vi "Consumer.vi"(8 "error in (no error)":errorcluster, 9 "Data":variant, 10 "Case ID":string, 11 "Guardian Subpanel in":refnum<class "Guardian Subpanel.lvclass">) -> (0 "error out":errorcluster, 3 "Guardian Subpanel out":refnum<class "Guardian Subpanel.lvclass">)   [LabVIEW 2026, in "TALOS.lvlib" / "Guardian Subpanel.lvlib" / "Guardian Subpanel.lvclass"]
uses:
  Guardian Subpanel.lvclass
  C:/LabVIEW Code/TALOS/talos/Father of all uServices/Father of all uServices/Father of all uServices.lvclass
  Guardian Subpanel Consumer Case Selector.ctl
  <vilib>/Utility/error.llb/DialogType.ctl
  Father of all uServices/Father of all uServices/Father of all uServices.lvclass/Father of all uServices.ctl
  Ancestor/Ancestor/Ancestor.lvclass/Ancestor.ctl
  <vilib>/AdvancedString/1D String Array to Delimited String (string).vi
  Support VIs/Substitute Error.vi
  Support VIs/Generate Error.vi
  FGV/Error Memory/Get Error Description.vi
  Support VIs/Get PC name.vi
  Ancestor/Ancestor/Read ID.vi
  Support VIs/Get Class Name.vi
  FGV/Error Memory/Error Memory Core.vi
  <vilib>/AdvancedString/Delimited String to 1D String Array.vi
  <vilib>/AdvancedString/Delimited String to 1D String Array (string).vi
  FGV/Error Memory/Error Crt Lvl checker.vi
  FGV/Error Memory/Error Memory Core.vi/40c8088d-b597-4017-91af-faa98e00292e.vi
  FGV/Error Memory/Error Memory Core.vi/d4a3ab98-063c-4e44-b43d-fbdcfe6c2be2.vi
  Support VIs/Global Memory.vi
  <vilib>/Utility/LVClass/Get LV Class Name.vi
  Support VIs/Is in Packed Library.vi
  Support VIs/TALOS Root path.vi
  Support VIs/Read CSV worksheet.vi
  Support VIs/Global Constants.vi
  <vilib>/Utility/error.llb/General Error Handler.vi
  Support VIs/Error Log.vi
  Ancestor/Ancestor/Ancestor.lvclass
  <vilib>/Comparison/Equal/Equal Functor/Equal Functor.lvclass
  Father of all uServices/Father of all uServices/Father of all uServices.lvclass
  TALOS.lvlib
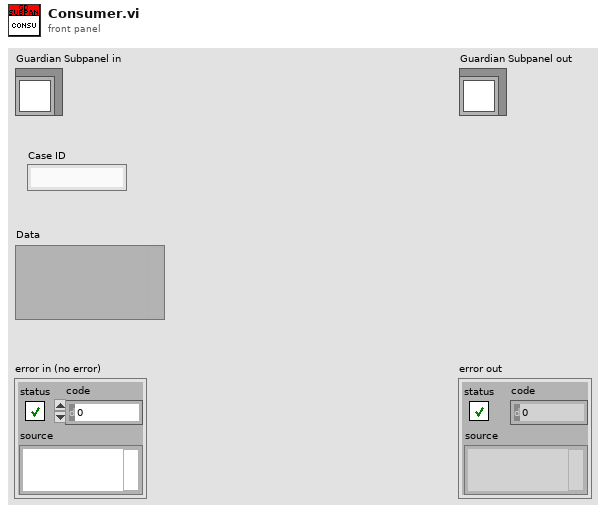
[diagram p1: front panel]
types:
  T1 = typedef "TALOS.lvlib/Guardian Subpanel.lvlib/Guardian Subpanel.lvclass/Guardian Subpanel Consumer Case Selector.ctl" = enum16{"uServices launchable", "Update Bearer"}
  T2 = typedef "DialogType.ctl" = u16
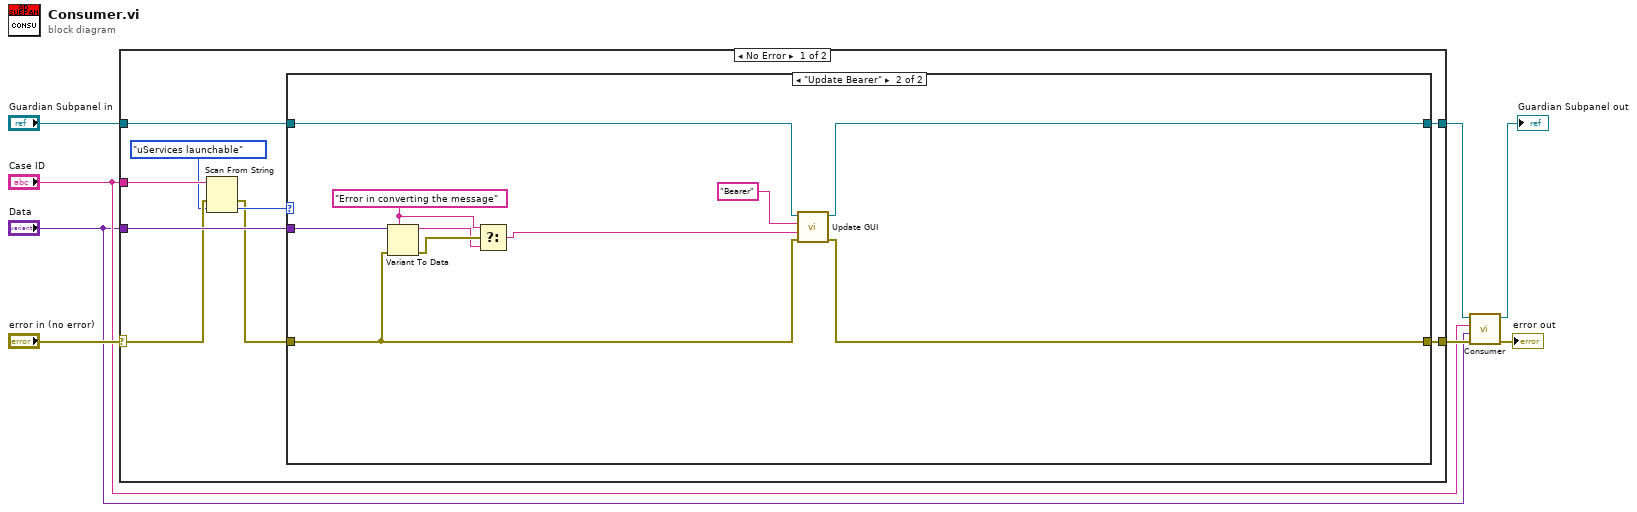
[diagram p0: block diagram]
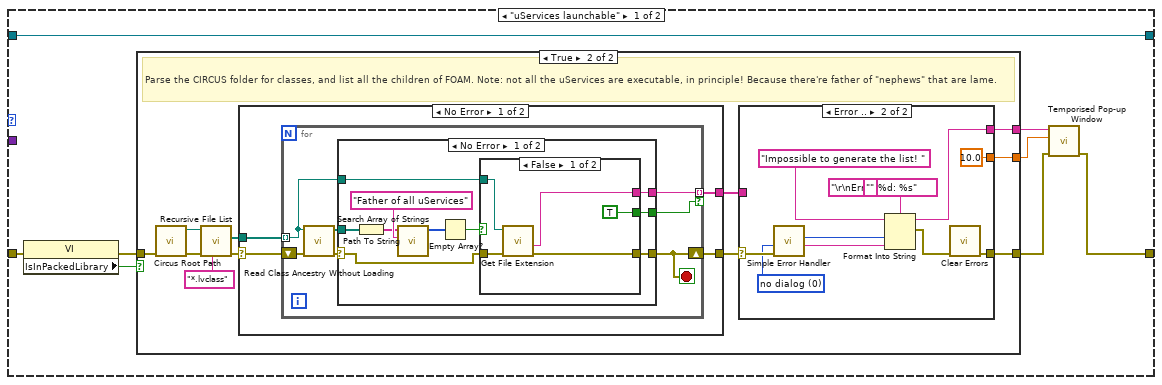
[diagram p2: hidden frame]
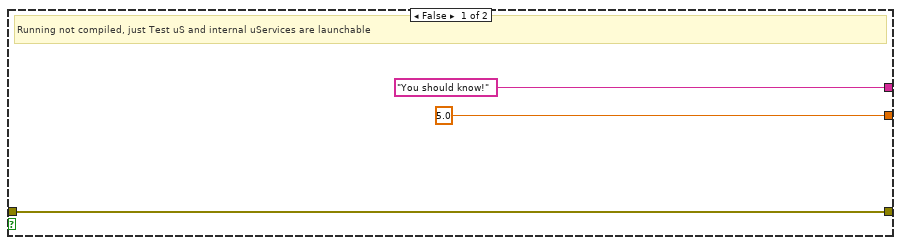
[diagram p3: hidden frame]
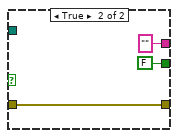
[diagram p4: hidden frame]
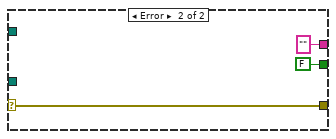
[diagram p5: hidden frame]
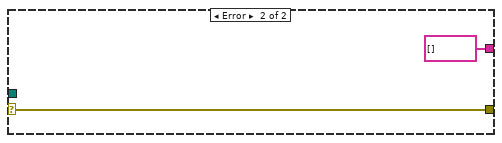
[diagram p6: hidden frame]
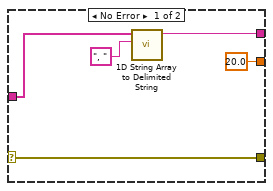
[diagram p7: hidden frame]
diagram:
  n1 = case shown="No Error" "error in (no error)" {
    selector: "error in (no error)" -> [w11 w99]
    tunnel: "Guardian Subpanel in" -> [w16 w100]
    tunnel: [w14 w100] -> w4
    tunnel: [w15 w99] -> w3
    tunnel: "Case ID" -> [w13 _]
    tunnel: "Data" -> [w17 _]
    frame No Error {
      n2 = Scan From String(input string=w13, error in=w11, default 1=Guardian_Subpanel_Consumer_Case_Selector."uServices launchable" ("Guardian Subpanel Consumer Case Selector")) -> (error out=w10:errorcluster, output 1=w12:T1)  [unwired: 2 in, 2 out]
      n3 = case shown="\"Update Bearer\"" w12 {
        tunnel: w17 -> [_ w98]
        tunnel: w10 -> [w23 w90]
        tunnel: w16 -> [w25 w96]
        tunnel: [w24 w89] -> w15
        tunnel: [w25 w97] -> w14
        frame "uServices launchable" {
          n4 = property class="VI"(error in=w23) -> (error out=w22:errorcluster, "IsInPackedLibrary"=w21:bool)  [unwired: 1 in, 1 out]
          n5 = case shown="True" w21 {
            tunnel: w22 -> [w26 w39]
            tunnel: ["You should know!" w33] -> w20
            tunnel: [5.0 w32] -> w19
            tunnel: [w26 w31] -> w18
            frame False {
              # "Running not compiled, just Test uS and internal uServices are launchable"
            }
            frame True {
              # "Parse the CIRCUS folder for classes, and list all the children of FOAM. Note: not all the uServices are executable, in principle! Because there're father of \"nephews\" that are lame."
              n6 = call "Circus Root Path.vi"("error in (no error)"=w39) -> ("error out"=w38:errorcluster, "Circus Root Path"=w37:path)  [unwired: 9 in]
              n7 = call <vilib>:"Recursive File List.vi"("pattern"="*.lvclass", "error in (no error)"=w38, "Folder Path"=w37) -> ("error out"=w35:errorcluster, "All Files in Dir"=w34:path[])  [unwired: 4 in, 3 out]
              n8 = case shown="No Error" w35 {
                selector: w35 -> [w43 w73]
                tunnel: w34 -> [w42 _]
                tunnel: [w41 w73] -> w30
                tunnel: [w40 string[] []] -> w29
                frame No Error {
                  n9 = for {
                    tunnel: w42 -> [w46] mode=indexing
                    shift-right: [w47] -> w41
                    shift-left: w43 -> [w50]
                    tunnel: [w45] -> w40 mode=indexing if=w44
                    stop <- w47 stop-if-true
                    n10 = call <vilib>:"Read Class Ancestry Without Loading.vi"("error in (no error)"=w50, "LabVIEW Class Path"=w46) -> ("error out"=w49:errorcluster, "Class Ancestry"=w48:path[])  [unwired: 8 in]
                    n11 = case shown="No Error" w49 {
                      selector: w49 -> [w54 w71]
                      tunnel: w48 -> [w60 _]
                      tunnel: [w53 w71] -> w47
                      tunnel: w46 -> [w55 _]
                      tunnel: [w52 ""] -> w45
                      tunnel: [w51 FALSE] -> w44
                      frame No Error {
                        n12 = Path To String(path=w60) -> (string=w58:string[])
                        n13 = call "Search Array of Strings.vi"("search string"="Father of all uServices", "Search array"=w58) -> ("indices"=w57:i32[])  [unwired: 8 in, 1 out]
                        n14 = Empty Array?(array=w57) -> (empty?=w56:bool)
                        n15 = case shown="False" w56 {
                          tunnel: w55 -> [w64 _]
                          tunnel: w54 -> [w65 w67]
                          tunnel: [w63 w67] -> w53
                          tunnel: [w62 ""] -> w52
                          tunnel: [TRUE FALSE] -> w51
                          frame False {
                            n16 = call <vilib>:"Get File Extension.vi"("error in (no error)"=w65, "file"=w64) -> ("error out"=w63:errorcluster, "filename without extension"=w62:string)  [unwired: 5 in, 3 out]
                          }
                          frame True {
                          }
                        }
                      }
                      frame Error {
                      }
                    }
                  }
                }
                frame Error {
                }
              }
              n17 = case shown="Error .." w30 {
                selector: w30 -> [w78 w88]
                tunnel: [w78 w82] -> w31
                tunnel: [w76 w81] -> w33
                tunnel: [20.0 10.0] -> w32
                tunnel: w29 -> [w77 _]
                frame No Error {
                  n18 = call-poly <vilib>:"1D String Array to Delimited String.vi"("delimiter"=", ", "string array"=w77) -> ("delimited string"=w76:string)  [unwired: 9 in]
                }
                frame Error {
                  (unwired) "\r\nError %d: %s" ("format string")
                  w87 = T2 0 items=["no dialog", "OK message", "continue or stop message", "OK message + warnings", "continue/stop + warnings"] ("type of dialog (OK msg:1)")
                  n19 = call <vilib>:"Simple Error Handler.vi"("type of dialog (OK msg:1)"=w87, "error in (no error)"=w88) -> ("code out"=w84:i32, "source out"=w85:string)  [unwired: 3 in, 3 out]
                  n20 = Format Into String(format string="", initial string="Impossible to generate the list! ", w84, w85) -> (resulting string=w81:string, error out=w83:errorcluster)  [unwired: 1 in]
                  n21 = call <vilib>:"Clear Errors.vi"("error in (no error)"=w83) -> ("error out"=w82:errorcluster)  [unwired: 5 in, 1 out]
                }
              }
            }
          }
          n22 = call "Temporised Pop-up Window.vi"("error in (no error)"=w18, "Timeout"=w19, "Text"=w20) -> ("error out"=w24:errorcluster)  [unwired: 8 in]
        }
        frame "Update Bearer" {
          w94 = "Error in converting the message"
          n23 = Variant To Data(error in=w90, type=w94, Variant=w98) -> (data=w93:string, error out=w95:errorcluster)
          n24 = Select(t=w94, s=w95, f=w93) -> (s? t:f=w92:string)
          n25 = call "Update GUI.vi"("error in (no error)"=w90, "Data"=w92, "GUI Item Name"="Bearer", "uService Template in"=w96) -> ("error out"=w89:errorcluster, "uService Template out"=w97:refnum<class "Guardian Subpanel.lvclass">)  [unwired: 6 in]
        }
      }
    }
    frame Error {
    }
  }
  n26 = call-parent "Consumer.vi"("error in (no error)"=w3, "Data"="Data", "Case ID"="Case ID", "uService Template in"=w4) -> ("error out"=→"error out":errorcluster, "uService Template out"=→"Guardian Subpanel out":refnum<class "Guardian Subpanel.lvclass">)  [unwired: 6 in]
